vi "GetHostName.vi"(4 "error in (no error)":errorcluster, 6 "DeviceKey In":string, 7 "CmdLib In":refnum<k24>) -> (0 "error out":errorcluster, 1 "Hostname":string, 2 "DeviceKey Out":string, 3 "CmdLib Out":refnum<k24>)   [LabVIEW 2009]
uses:
  C:/Code/Apps/Utilities/Picomotor/PicomotorApp/Install/Samples/LabVIEW/Model 8742/LabVIEW 2009/CmdLib.dll
panel:
  in  "name":string
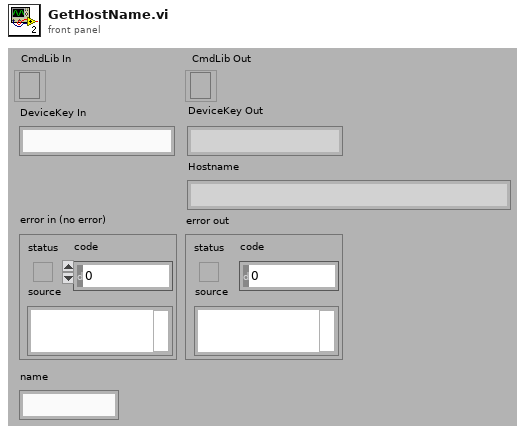
[diagram p1: front panel]
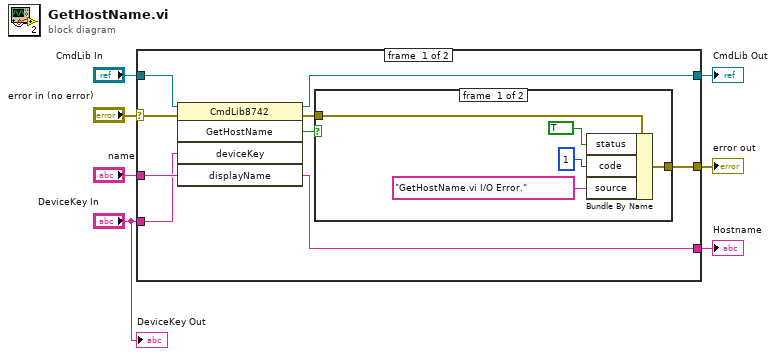
[diagram p0: block diagram]
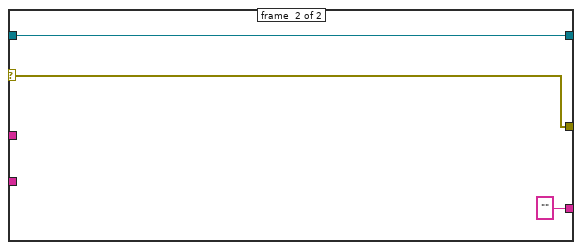
[diagram p3: hidden frame]
diagram:
  n1 = case shown="No Error" "error in (no error)" {
    selector: "error in (no error)" -> [w11 w23]
    tunnel: "CmdLib In" -> [w16 w25]
    tunnel: [w15 w25] -> w6
    tunnel: "name" -> [w14 _]
    tunnel: [w13 "" ("identification")] -> w4
    tunnel: "DeviceKey In" -> [w12 _]
    tunnel: [w8 w23] -> w1
    frame #0 {
      n2 = invoke class="CmdLib8742" method="GetHostName"(reference=w16, error in=w11, "deviceKey"=w12, "displayName"=w14) -> (reference out=w15:refnum<k24>, error out=w9:errorcluster, "GetHostName"=w10:bool, "displayName"=w13:string)  [unwired: 1 in, 1 out]
      n3 = case shown="False" w10 {
        tunnel: w9 -> [w21 w22]
        tunnel: [w20 w22] -> w8
        frame #0 {
          n4 = Bundle By Name(cluster=w21, "status"=TRUE, "code"=1, "source"="GetHostName.vi I/O Error.") -> (w20:errorcluster)
        }
        frame #1 {
        }
      }
    }
    frame #1 {
    }
  }
  "error out" <- w1
  "CmdLib Out" <- w6
  "Hostname" <- w4
  "DeviceKey Out" <- "DeviceKey In"
